vi "RECenterROI (SubVI).vi"(1 "Image in":T1, 7 "ROI in LTRB":i32[](array[numeric]), 12 "error out 2":errorcluster) -> (3 "Imageout":u8[][](array[numeric]), 10 "LTRB improved":u32[](array[numeric]), 14 "error out":errorcluster)   [LabVIEW 2011]
uses:
  <vilib>/vision/Image Controls.llb/IMAQ Image.ctl
panel:
  out "centered":u8[][](graph)
  out "original":u8[][](graph)
  out "Coordinates (pix)":dbl[](array[numeric]) format="%.2f"
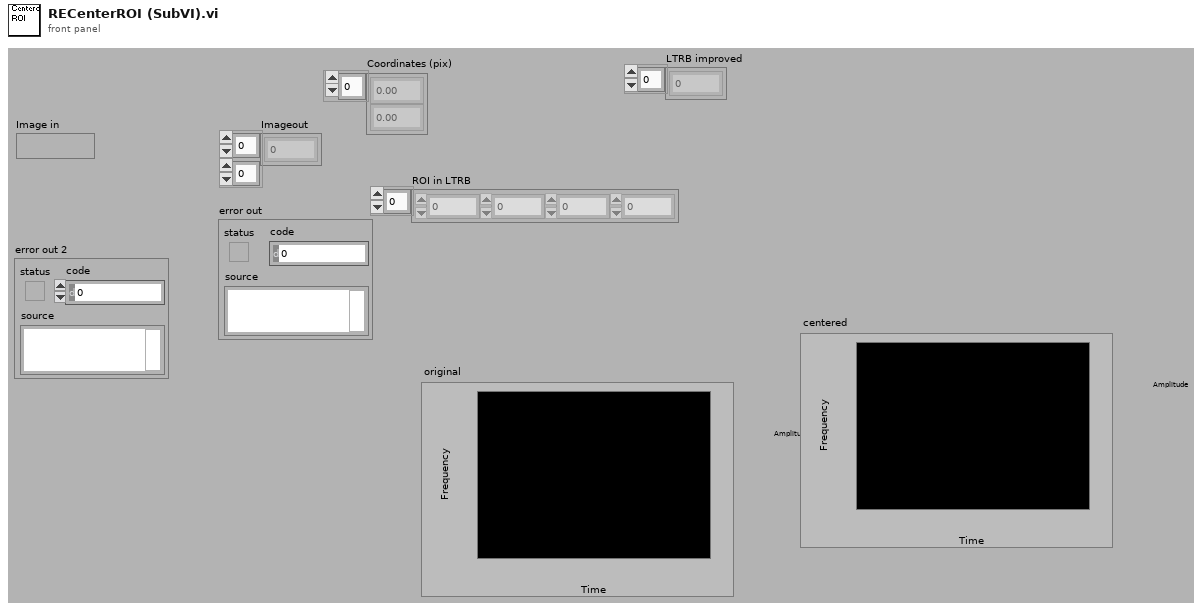
[diagram p1: front panel]
types:
  T1 = typedef "IMAQ Image.ctl" = refnum<image>
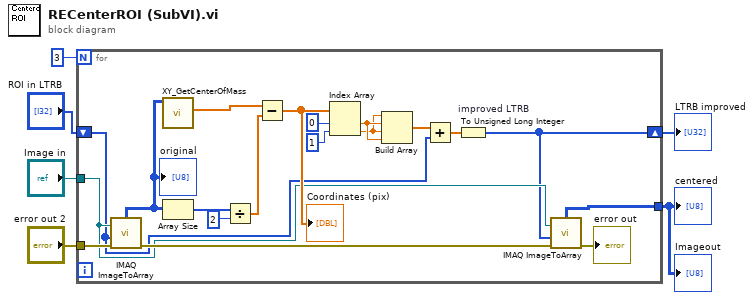
[diagram p0: block diagram]
diagram:
  n1 = for {
    N: 3 -> [_]
    tunnel: "error out 2" -> [w25]
    tunnel: "Image in" -> [w13]
    tunnel: [w10] -> w3
    shift-right: [w12] -> w4
    shift-left: "ROI in LTRB" -> [w7]
    n2 = call "IMAQ ImageToArray"("error in (no error)"=w25, "Optional Rectangle"=w7, "Image"=w13) -> ("error out"=w15:errorcluster, "Image Pixels (U8)"=w11:u8[][])  [unwired: 4 out]
    "original" <- w11
    n3 = call "XY_GetCenterOfMass.vi"("Image in"=w11) -> ("corner-based Coordinates (pix)"=w21:dbl[])  [unwired: 9 out]
    n4 = Array Size(array=w11) -> (size(s)=w24:i32[])
    n5 = Divide(x=w24, y=2) -> (x/y=w22:dbl[])
    n6 = Subtract(x=w21, y=w22) -> (x-y=w20:dbl[])
    "Coordinates (pix)" <- w20
    n7 = Index Array(array=w20, index #1=0 ("index"), index #2=1 ("index")) -> (element #1=w9:dbl, element #2=w8:dbl)
    n8 = Build Array(w8, w9, w8, w9) -> (w17:dbl[])
    n9 = Add(x=w17, y=w7) -> (x+y=w16:dbl[])
    n10 = To Unsigned Long Integer "improved LTRB"(number=w16) -> (unsigned 32bit integer=w12:u32[])
    n11 = call "IMAQ ImageToArray"("error in (no error)"=w15, "Optional Rectangle"=w12, "Image"=w13) -> ("error out"=→"error out":errorcluster, "Image Pixels (U8)"=w10:u8[][])  [unwired: 4 out]
  }
  "Imageout" <- w3
  "centered" <- w3
  "LTRB improved" <- w4
